vi "test -- PLL analyzer V1.vi"() -> ()   [LabVIEW 2017]
uses:
  lorentzian.ctl
  circle corners.ctl
  pid -- parameters.ctl
  <vilib>/event_ctls.llb/eventvkey.ctl
  cursor winow.ctl
  agregator -- action.ctl
  cursor window action.ctl
  four-corner circle transformation.ctl
  cursor action.ctl
  publisher action.ctl
  Q -- check range -- i -- real.vi
  draw a line.vi
  draw a circle.vi
  linear interpolation - real.vi
  linear interpolation iiii- complex.vi
  Q - not nan -- real.vi
  generate linear region.vi
panel:
  in  "all 3":enum32{"all", "other"}(tab)
  in  "total exp time (sec)":dbl=200.0 format="%#_10f"
  in  "total number of points":dbl=50000.0 format="%#_10f"
  out "dt (sec)":dbl=0.004 format="%#_10f"
  out "Plot: complex plane - filter":cluster{dbl[], dbl[]}[](graph)=[{[0.3333333333333333, 0.3330409433662861, 0.3321642864165014, 0.33070490043815925, 0.3286653456901683, 0.3260492002446019, 0.32286105370954366, 0.31910649917735573, 0.3147921234124937, 0.3099254952960838, 0.3045151525475336, 0.29857058674647097, 0.2921022266812878, 0.28512142005350216, 0.27764041357003316, 0.2696723314583158, 0.2612311524419466, 0.25233168521725213, 0.24298954247380383, 0.23322111350445518, 0.22304353545295275, 0.21247466324956327, 0.2015330382874583, 0.1902378558948106, 0.17860893165966557, 0.16666666666666669, 0.15443201170662058, 0.14192643052169093, 0.12917186215070103, 0.1161906824406051, 0.10300566479164915, 0.08963994020508864, 0.07611695670355195, 0.06246043819524158, 0.04869434285413729, 0.03484282108921789, 0.02093017317643784, 0.006980806627785684, -0.0069808066277855674, -0.020930173176437725, -0.034842821089217775, -0.0486943428541371, -0.062460438195241455, -0.07611695670355184, -0.08963994020508853, -0.10300566479164903, -0.116190682440605, -0.12917186215070092, -0.14192643052169077, -0.1544320117066205, -0.16666666666666657, -0.17860893165966546, -0.19023785589481051, -0.20153303828745828, -0.21247466324956313, -0.22304353545295263, -0.23322111350445507, -0.24298954247380378, -0.2523316852172521, -0.26123115244194656, -0.26967233145831576, -0.27764041357003305, -0.2851214200535021, -0.29210222668128777, -0.29857058674647086, -0.3045151525475336, -0.30992549529608376, -0.31479212341249363, -0.3191064991773557, -0.32286105370954366, -0.3260492002446018, -0.32866534569016825, -0.33070490043815925, -0.3321642864165014, -0.3330409433662861, -0.3333333333333333, -0.3330409433662861, -0.3321642864165014, -0.33070490043815925, -0.3286653456901683, -0.3260492002446019, -0.3228610537095437, -0.3191064991773558, -0.31479212341249374, -0.3099254952960838, -0.3045151525475337, -0.29857058674647097, -0.2921022266812879, -0.2851214200535023, -0.2776404135700333, -0.26967233145831593, -0.2612311524419467, -0.25233168521725224, -0.24298954247380392, -0.2332211135044552, -0.2230435354529528, -0.21247466324956338, -0.20153303828745844, -0.1902378558948107, -0.17860893165966568, -0.1666666666666668, -0.1544320117066207, -0.14192643052169096, -0.12917186215070106, -0.11619068244060515, -0.10300566479164919, -0.0896399402050886, -0.07611695670355222, -0.06246043819524183, -0.04869434285413747, -0.03484282108921807, -0.02093017317643803, -0.006980806627785872, 0.006980806627785453, 0.02093017317643761, 0.03484282108921766, 0.04869434285413707, 0.06246043819524142, 0.07611695670355181, 0.08963994020508849, 0.10300566479164908, 0.11619068244060474, 0.1291718621507007, 0.1419264305216906, 0.1544320117066203, 0.16666666666666644, 0.17860893165966532, 0.19023785589481038, 0.2015330382874581, 0.2124746632495631, 0.22304353545295258, 0.233221113504455, 0.24298954247380372, 0.252331685217252, 0.2612311524419465, 0.26967233145831576, 0.27764041357003294, 0.28512142005350205, 0.2921022266812877, 0.2985705867464708, 0.3045151525475335, 0.3099254952960837, 0.3147921234124936, 0.3191064991773557, 0.32286105370954366, 0.3260492002446018, 0.32866534569016825, 0.33070490043815925, 0.3321642864165014, 0.3330409433662861], [-0.3333333333333333, -0.31937478209026676, -0.30544071888922814, -0.2915555888118986, -0.27774375109463256, -0.2640294363940802, -0.2504367042783817, -0.23698940101850946, -0.2237111177538056, -0.21062514910510735, -0.1977544523080666, -0.1851216069383575, -0.17274877529942825, -0.16065766354228994, -0.148869483585552, -0.13740491590250895, -0.12628407324056323, -0.11552646533663152, -0.10515096469043711, -0.09517577345573225, -0.08561839150753528, -0.07649558574140364, -0.06782336065860123, -0.05961693028876536, -0.051890691499328345, -0.04465819873852045, -0.03793214025626174, -0.03172431584466018, -0.026045616137166494, -0.02090600350270283, -0.016314494568282156, -0.01227914440078065, -0.008807032375613255, -0.005904249757103797, -0.003575889012337241, -0.0018260348772422552, -0.000657757190576147, -7.310550838485197e-05, -7.310550838485197e-05, -0.000657757190576147, -0.0018260348772421997, -0.003575889012337241, -0.005904249757103741, -0.008807032375613255, -0.012279144400780595, -0.0163144945682821, -0.02090600350270283, -0.02604561613716644, -0.03172431584466012, -0.03793214025626174, -0.04465819873852045, -0.05189069149932829, -0.0596169302887653, -0.06782336065860123, -0.07649558574140353, -0.08561839150753517, -0.09517577345573214, -0.10515096469043705, -0.11552646533663147, -0.12628407324056315, -0.13740491590250892, -0.14886948358555185, -0.16065766354228977, -0.17274877529942811, -0.18512160693835739, -0.19775445230806651, -0.21062514910510727, -0.22371111775380553, -0.2369894010185093, -0.2504367042783816, -0.26402943639408005, -0.27774375109463245, -0.29155558881189847, -0.3054407188892281, -0.3193747820902667, -0.33333333333333315, -0.3472918845763997, -0.3612259477774383, -0.37511107785476794, -0.38892291557203396, -0.40263723027258636, -0.4162299623882848, -0.429677265648157, -0.4429555489128609, -0.45604151756155914, -0.4689122143585999, -0.481545059728309, -0.4939178913672383, -0.5060090031243767, -0.5177971830811146, -0.5292617507641575, -0.5403825934261033, -0.551140201330035, -0.5615157019762295, -0.5714908932109344, -0.5810482751591313, -0.5901710809252629, -0.5988433060080653, -0.6070497363779013, -0.6147759751673383, -0.6220084679281461, -0.6287345264104047, -0.6349423508220065, -0.6406210505295, -0.6457606631639639, -0.6503521720983845, -0.6543875222658859, -0.6578596342910533, -0.6607624169095627, -0.6630907776543293, -0.6648406317894244, -0.6660089094760905, -0.6665935611582818, -0.6665935611582818, -0.6660089094760905, -0.6648406317894244, -0.6630907776543293, -0.6607624169095629, -0.6578596342910534, -0.654387522265886, -0.6503521720983845, -0.6457606631639639, -0.6406210505295002, -0.6349423508220067, -0.628734526410405, -0.6220084679281463, -0.6147759751673385, -0.6070497363779015, -0.5988433060080656, -0.5901710809252632, -0.5810482751591315, -0.5714908932109346, -0.5615157019762296, -0.5511402013300353, -0.5403825934261035, -0.5292617507641577, -0.517797183081115, -0.506009003124377, -0.4939178913672387, -0.4815450597283094, -0.4689122143586003, -0.45604151756155953, -0.44295554891286126, -0.4296772656481574, -0.4162299623882851, -0.4026372302725866, -0.38892291557203423, -0.3751110778547682, -0.3612259477774386, -0.3472918845764]}, {[0.0, 0.0, 0.0, 0.0, 0.0, 0.0, 0.0, 0.0, 0.0, 0.0, 0.0, 0.0, 0.0, 0.0, 0.0, 0.0, 0.0, 0.0, 0.0, 0.0], [0.0, -0.03333333333333333, -0.06666666666666667, -0.1, -0.13333333333333333, -0.16666666666666666, -0.2, -0.23333333333333334, -0.26666666666666666, -0.3, -0.3333333333333333, -0.36666666666666664, -0.4, -0.43333333333333335, -0.4666666666666667, -0.5, -0.5333333333333333, -0.5666666666666667, -0.6, -0.6333333333333333]}, {[0.3333333333333333, 0.3, 0.26666666666666666, 0.2333333333333333, 0.19999999999999998, 0.16666666666666666, 0.1333333333333333, 0.09999999999999998, 0.06666666666666665, 0.033333333333333326, 0.0, -0.033333333333333326, -0.06666666666666671, -0.10000000000000003, -0.13333333333333336, -0.16666666666666669, -0.2, -0.23333333333333334, -0.26666666666666666, -0.3], [-0.3333333333333333, -0.3333333333333333, -0.3333333333333333, -0.3333333333333333, -0.3333333333333333, -0.3333333333333333, -0.3333333333333333, -0.3333333333333333, -0.3333333333333333, -0.3333333333333333, -0.3333333333333333, -0.3333333333333333, -0.3333333333333333, -0.3333333333333333, -0.3333333333333333, -0.3333333333333333, -0.3333333333333333, -0.3333333333333333, -0.3333333333333333, -0.3333333333333333]}]
  out "zi frreq":dbl=953.6192037473343 format="%#_5f"
  in  "PID parameters":T1={"P (sec)"=0.07054802310718643, "I (sec)"=0.2727272727272727}
  in  "visc hist time (sec)":dbl=5.0 format="%#_10f"
  out "dev frreq":dbl=952.9395994616418 format="%#_5f"
  out "off freq":dbl=0.6796042856924487 format="%#_5f"
  in  "I (sec)":dbl(slide)=0.2727272727272727 scale=0.0..3.0
  in  "P (sec)":dbl(slide)=0.07054802310718643 scale=0.001..1.0
  out "circle lorentzian":T2={"Amplitude"=1.0, "omega(0)"=1000.0, "Gamma"=3.0, "phase"=0.0, "Q"=300.0, "Norm  Ampl"=nan, "z (inf)"=0.0+0.0i, "4corners"={"z (-pi/2)"=9.277908004825974e-07+0.0007240755403629966i, "z(inf)"=2.6527949823343002e-05+0.0007477540585896028i, "z (pi/2)"=2.8494315967368497e-06+0.0007733542176124632i, "z center"=1.8886111986097237e-06+0.0007487148789877299i, "z(0)"=-2.2750727426123552e-05+0.000749675699385857i, "radius"=2.4658065287076567e-05}} {"z (inf)" format="%#9_9f"; "Q" format="%#9_9f"; "phase" format="%#9_9f"; "Gamma" format="%#9_9f"; "omega(0)" format="%#9_9f"}
  in  "cursor bracket: fit boundaries":T4={"left"=395.0, "right "=505.0, "center"=450.0, "window"=110.0, "cursors"=[0, 1, 2], "relative"=0, "absolute"=0, "fixed vertical offset"=0.0, "vertical offset"=0.0, "skew"=0.0, "default window frac"=0.1, "kind"=enum."symmetric", "skew.left"=0.5, "skew.right"=0.5, "Plot ref"=refnum, "wing order"=enum."forw"}
  out "VKey":T5=enum."Cmd"
  out "Char":i16
  in  "lorentzian -- basic":T2={"Amplitude"=1.0, "omega(0)"=1000.0, "Gamma"=3.0, "phase"=0.0, "Q"=300.0, "Norm  Ampl"=nan, "z (inf)"=0.0+0.0i, "4corners"={"z (-pi/2)"=9.277908004825974e-07+0.0007240755403629966i, "z(inf)"=2.6527949823343002e-05+0.0007477540585896028i, "z (pi/2)"=2.8494315967368497e-06+0.0007733542176124632i, "z center"=1.8886111986097237e-06+0.0007487148789877299i, "z(0)"=-2.2750727426123552e-05+0.000749675699385857i, "radius"=2.4658065287076567e-05}} {"z (inf)" format="%#9_9f"; "Q" format="%#9_9f"; "phase" format="%#9_9f"; "Gamma" format="%#9_9f"; "omega(0)" format="%#9_9f"}
  in  "all 2":enum32{"all", "other"}(tab)
  out "Plot: circle sweep window":cluster{dbl[], dbl[]}[](graph)
  out "dev out":cdb=0.2506043041344095-0.553125493931521i format="%#_10f"
  out "time(sec)":dbl=179.1847980649909 format="%#_5f"
  in  "all":enum32{"all", "other"}(tab)
  out "Plot: hist":cluster{"all rows":dbl[], "all rows":dbl[]}[](graph)
  out "center freq (Hz)":dbl=-0.35260838541595674
  out "window  (Hz)":dbl=17.234446484426172
  out "left freq (Hz)":dbl=-8.969831627629043
  out "right freq (Hz)":dbl=8.26461485679713
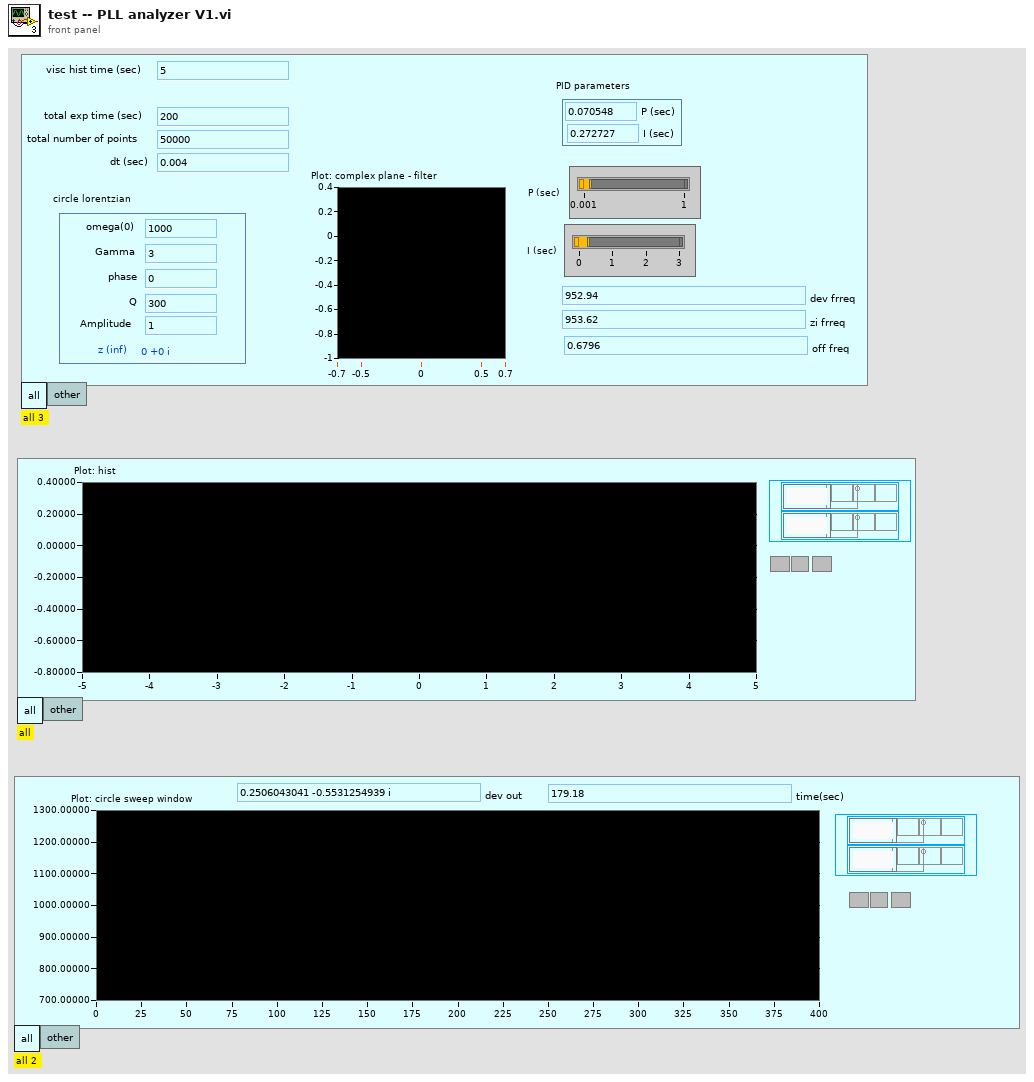
[diagram p1: front panel]
types:
  T1 = typedef "pid -- parameters.ctl" = cluster{"P (sec)":dbl, "I (sec)":dbl}
  T2 = typedef "lorentzian.ctl" = cluster{"Amplitude":dbl, "omega(0)":dbl, "Gamma":dbl, "phase":dbl, "Q":dbl, "Norm  Ampl":dbl, "z (inf)":cdb, "4corners":T3}
  T3 = typedef "circle corners.ctl" = cluster{"z (-pi/2)":cdb, "z(inf)":cdb, "z (pi/2)":cdb, "z center":cdb, "z(0)":cdb, "radius":dbl}
  T4 = typedef "cursor winow.ctl" = cluster{"left":dbl, "right ":dbl, "center":dbl, "window":dbl, "cursors":i32[], "relative":i32, "absolute":i32, "fixed vertical offset":dbl, "vertical offset":dbl, "skew":dbl, "default window frac":dbl, "kind":enum16{"symmetric", "skewed", "fancy"}, "skew.left":dbl, "skew.right":dbl, "Plot ref":refnum<vi>, "wing order":enum16{"forw", "back"}}
  T5 = typedef "eventvkey.ctl" = enum16{"ASCII", "Enter", "Return", "Shift", "Ctrl", "Alt", "Cmd", "Opt", "Caps", "NumLock", "Clear", "Break", "Up", "Down", "Left", "Right", "Insert", "Delete", "Home", "End", "PageUp", "PageDown", "Escape", "Help", "Pause", "ScrollLock", "F1", "F2", "F3", "F4", "F5", "F6", "F7", "F8", "F9", "F10", "F11", "F12", "F13", "F14", "F15", "F16", "F17", "F18", "F19", "F20", "F21", "F22", "F23", "F24", "Play", "VolumeUp", "VolumeDown", "Mute", "Two Byte Char"}
  T6 = typedef "cursor window action.ctl" = enum16{"balance", "h. offset change", "cursor moves", "change center", "change window", "init", "check", "reset", "set y to middle", "idle", "-write all Y", "-write left.X", "-write center.X", "-write right.X", "-write all X", "-change center", "-change window", "-change skew", "-read cursor 2", "-read cursor 1", "-read cursor 0", "-read all cursors", "-reset", "-read plot scale", "-set y to middle", "-Q: center.Y is visible", "-Q: window is visible", "-parse center.Y", "-right left from center", "-left move", "-right move", "-set center.Y", "-empty", "-set cursors to default", "-check", "-write center.Y", "-copy cursor 1", "-copy cursor 0", "-copy cursor 2", "move right", "move left", "shrink", "broaden", "skew up", "skew down", "-write plot scale", "zoom X", "change cen&win", "zoom to all data", "color--red", "color--green", "color--yellow", "read", "zoom out", "zoom in", "slide right", "slide left"}
  T7 = typedef "agregator -- action.ctl" = enum16{"append", "interpolate", "empty!", "force", "init", "scale", "read last"}
  T8 = typedef "publisher action.ctl" = enum16{"set", "get"}
  T9 = typedef "cursor action.ctl" = enum16{"range", "read", "write", "check", "zoom out", "smart zoom out"}
  T10 = typedef "four-corner circle transformation.ctl" = enum16{"z(c) z(inf)", "z(c) z(zero)", "fix phase", "calculate lorentzian", "z(0) z(+-pi/2)", "shift to zcenter", "to  canonical", "get canonical phase", "get4corners"}
  T11 = typedef "interpolation state - complex.ctl" = cluster{"requested size":i32, "Array":cdb[], "actual number of elements":i32}
  T12 = typedef "interpolation state - real.ctl" = cluster{"requested size":i32, "Array":dbl[], "actual number of elements":i32}
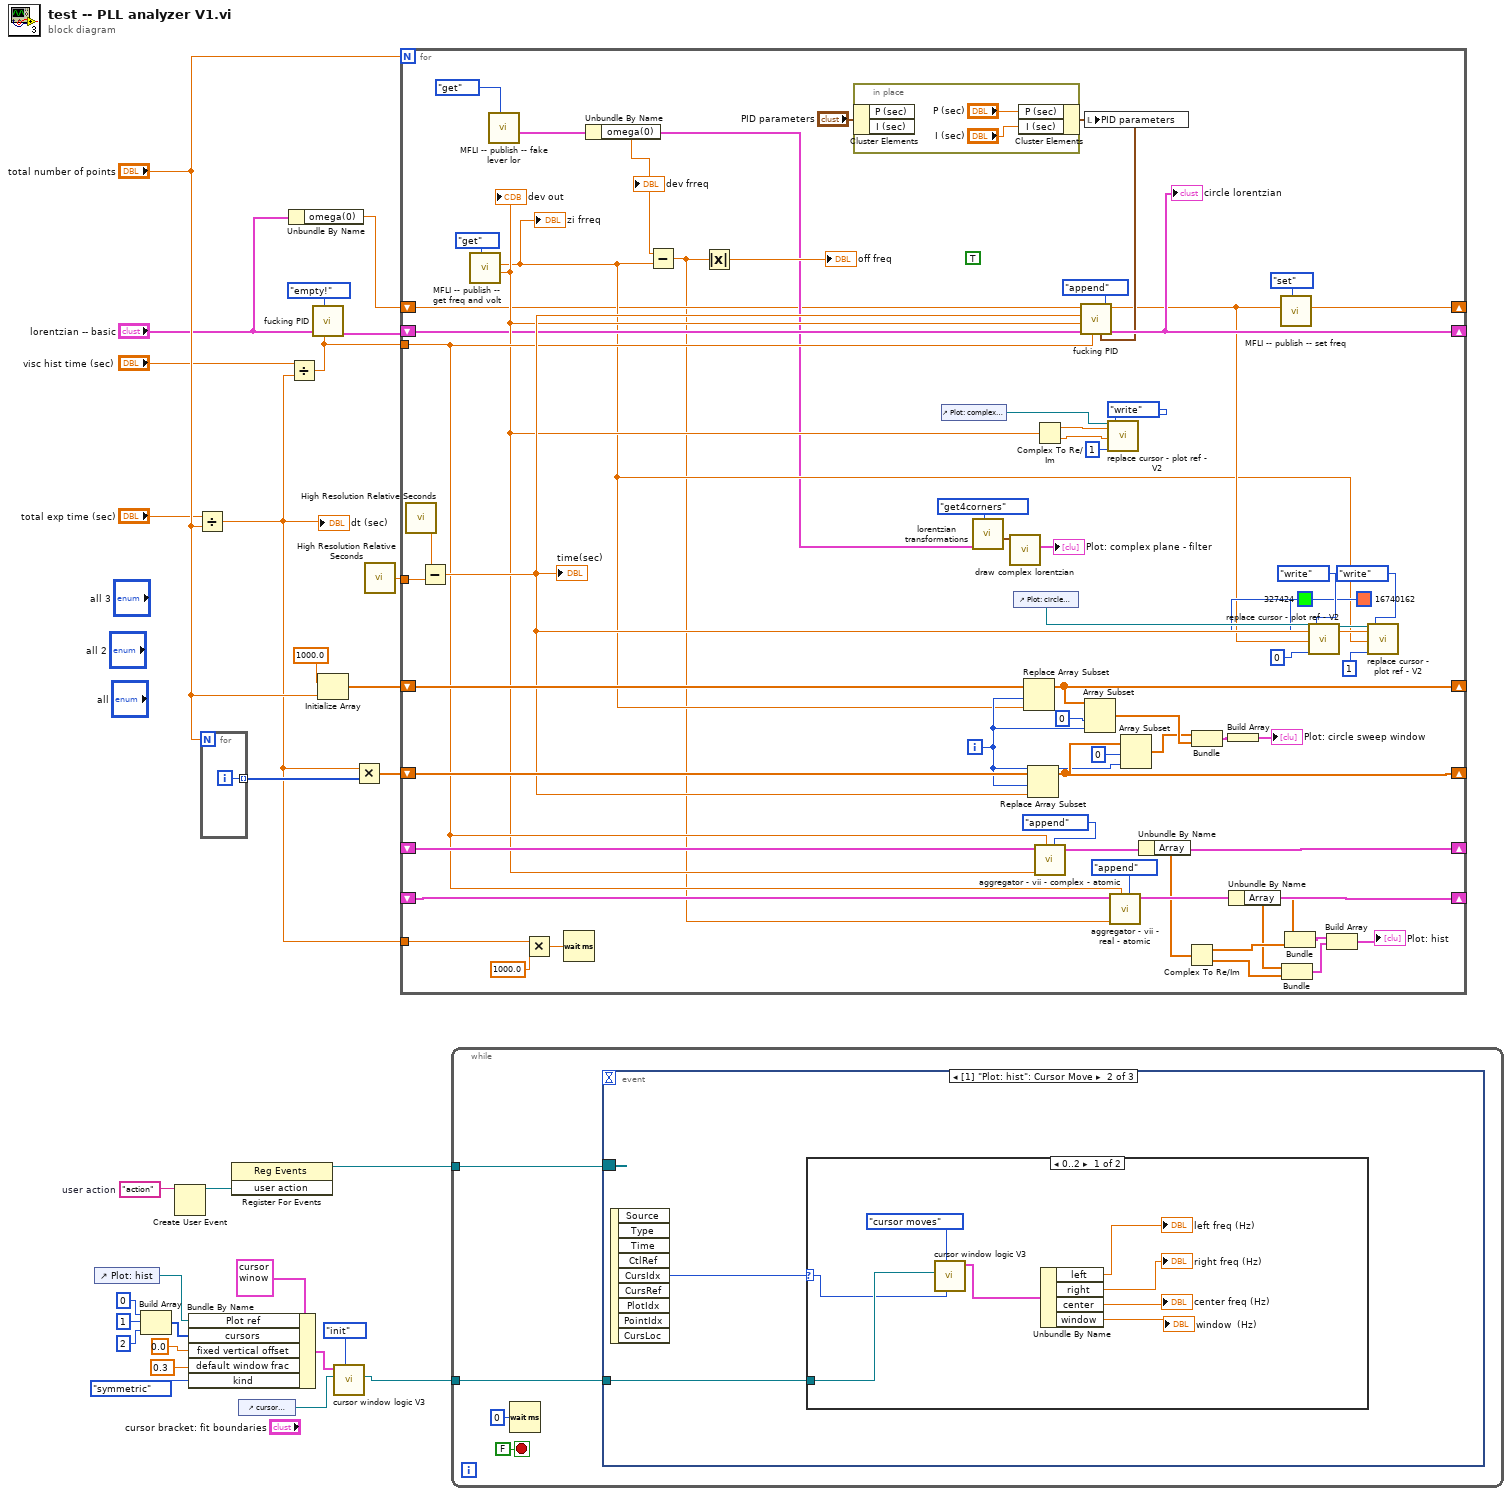
[diagram p0: block diagram]
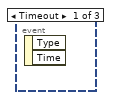
[diagram p2: hidden frame]
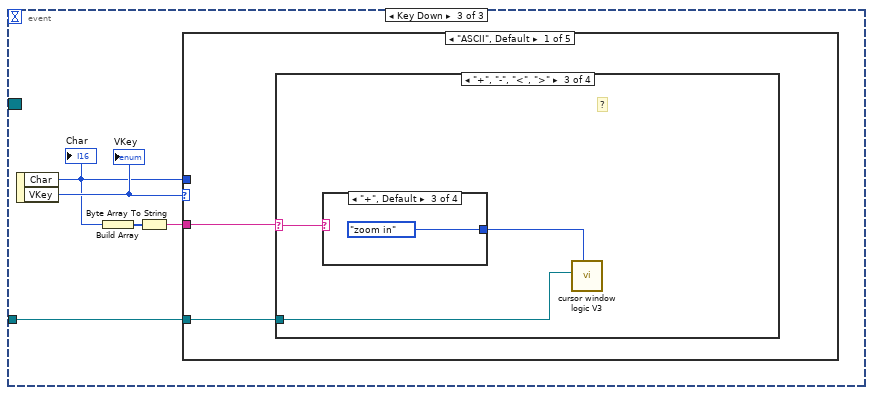
[diagram p4: hidden frame]
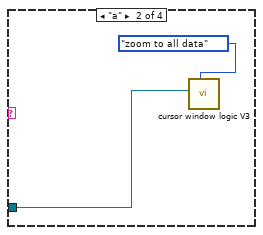
[diagram p6: hidden frame]
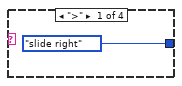
[diagram p7: hidden frame]
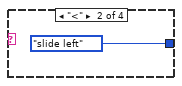
[diagram p8: hidden frame]
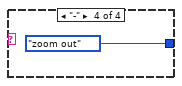
[diagram p9: hidden frame]
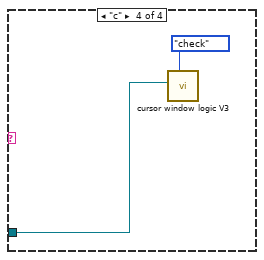
[diagram p10: hidden frame]
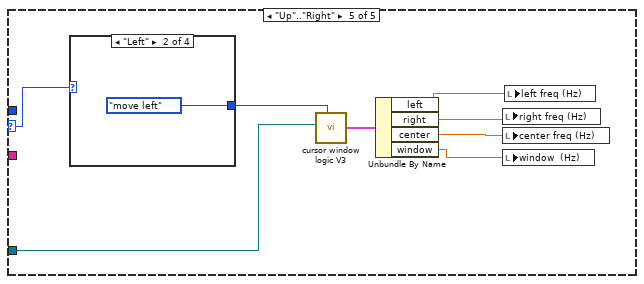
[diagram p14: hidden frame]
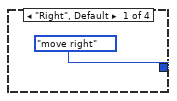
[diagram p15: hidden frame]
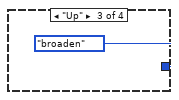
[diagram p16: hidden frame]
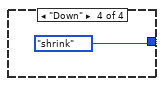
[diagram p17: hidden frame]
diagram:
  w18 = "action"  # user action
  n1 = control-ref of="Plot: hist"() -> (w16:refnum<vi>)
  n2 = Build Array(0, 1, 2) -> (w5:i32[])
  n3 = Create User Event(user event datatype=w18) -> (user event=w19:refnum<user-event>)  [unwired: 1 in, 1 out]
  n4 = Bundle By Name(cluster=T4 {"left"=0.0, "right "=0.0, "center"=0.0, "window"=0.0, "cursors"=[], "relative"=0, "absolute"=0, "fixed vertical offset"=0.0, "vertical offset"=0.0, "skew"=0.0, "default window frac"=0.0, "kind"=enum."symmetric", "skew.left"=0.0, "skew.right"=0.0, "Plot ref"=refnum, "wing order"=enum."forw"} ("cursor bracket: All, data window"), "Plot ref"=w16, "cursors"=w5, "fixed vertical offset"=0.0, "default window frac"=0.3 ("fixed vertical offset"), "kind"=enum16{"symmetric", "skewed", "fancy"}."symmetric") -> (w13:T4)
  n5 = Divide(x="total exp time (sec)", y="total number of points") -> (x/y=w24:dbl)
  "dt (sec)" <- w24
  n6 = for {
    N: "total number of points" -> [_]
    tunnel: [w31] -> w26 mode=indexing
    i -> [w31]
  }
  n7 = register-events(w19) -> (reference out=w17:refnum<event-registration>)  [unwired: 2 in, 1 out]
  n8 = control-ref of="cursor bracket: fit boundaries"() -> (w15:refnum<vi>)
  n9 = Unbundle By Name("lorentzian -- basic") -> ("omega(0)"=w1:dbl)
  n10 = Divide(x="visc hist time (sec)", y=w24) -> (x/y=w21:dbl)
  n11 = call "fucking PID.vi"("requested size"=w21, "PID action"=agregator_--_action."empty!", "lorentzian IN"="lorentzian -- basic") -> ("lorentzian  OUT"=w3:T2)  [unwired: 5 in, 3 out]
  n12 = Initialize Array(1000.0, "total number of points") -> (w29:dbl[])
  n13 = call "cursor window logic V3.vi"("cursor window action"=cursor_window_action."init", "cursor window in"=w15, "cursor window init"=w13) -> ("cursor window out"=w20:refnum<vi>)  [unwired: 7 in, 1 out]
  n14 = Multiply(x=w24, y=w26) -> (x*y=w25:dbl[])
  n15 = call <vilib>:"High Resolution Relative Seconds.vi"() -> ("relative seconds"=w30:dbl)
  n16 = for {
    N: "total number of points" -> [_]
    tunnel: w30 -> [w95]
    shift-right: [w73] -> _
    shift-left: w29 -> [w94]
    shift-right: [w69] -> _
    shift-left: w25 -> [w93]
    tunnel: w24 -> [w90]
    tunnel: w21 -> [w51]
    shift-right: [w62] -> _
    shift-left: w3 -> [w39]
    shift-right: [w47] -> _
    shift-left: _ -> [w55]
    shift-right: [w49] -> _
    shift-left: _ -> [w52]
    shift-right: [w34] -> _
    shift-left: w1 -> [w33]
    i -> [w67]
    (unwired) TRUE
    n17 = call <vilib>:"High Resolution Relative Seconds.vi"() -> ("relative seconds"=w92:dbl)
    n18 = Subtract(x=w92, y=w95) -> (x-y=w65:dbl)
    "time(sec)" <- w65
    n19 = call "MFLI -- publish -- get freq and volt.vi"("publisher action"=publisher_action."get") -> ("Voltage out (V)"=w42:cdb, "freq out (Hz)"=w38:dbl)  [unwired: 9 in]
    "dev out" <- w42
    "zi frreq" <- w38
    n20 = call "MFLI -- publish -- fake lever lor.vi"("publisher action"=publisher_action."get") -> ("lorentzian OUT"=w35:T2)  [unwired: 10 in]
    n21 = Multiply(x=w90, y=1000.0) -> (x*y=w91:dbl)
    n22 = Wait (ms)(milliseconds to wait=w91) -> ()  [unwired: 1 out]
    n23 = Unbundle By Name(w35) -> ("omega(0)"=w36:dbl)
    "dev frreq" <- w36
    n24 = Subtract(x=w36, y=w38) -> (x-y=w32:dbl)
    n25 = Absolute Value(x=w32) -> (abs(x)=→"off freq":dbl)
    n26 = in-place {
      n27 = in-place-cluster #1("PID parameters") -> ()  [unwired: 2 out]
      n28 = in-place-cluster #1("P (sec)"="P (sec)", "I (sec)"="I (sec)") -> (w44:T1)
    }
    n29 = control-ref of="Plot: complex plane - filter"() -> (w81:refnum<vi>)
    n30 = call "lorentzian transformations.vi"("4 corner circle transformation"=four-corner_circle_transformation."get4corners", "lorentzian in"=w35) -> ("4corners our"=w88:T3)  [unwired: 7 in, 2 out]
    n31 = call "draw complex lorentzian.vi"("4 corners"=w88) -> ("fancy circles"=→"Plot: complex plane - filter":cluster{dbl[], dbl[]}[])  [unwired: 10 in]
    n32 = control-ref of="Plot: circle sweep window"() -> (w74:refnum<vi>)
    n33 = Replace Array Subset(array=w94, new element=w38, index=w67) -> (w73:dbl[])
    n34 = Replace Array Subset(array=w93, new element=w65, index=w67) -> (w69:dbl[])
    n35 = Complex To Re/Im(x + iy=w42) -> (x=w83:dbl, y=w82:dbl)
    n36 = call "aggregator - vii - complex - atomic.vi"("aggregator action"=agregator_--_action."append", "requested size"=w51, "number"=w42, "state IN"=w55) -> ("state OUT"=w47:T11)  [unwired: 4 in, 3 out]
    n37 = call "fucking PID.vi"("PID parameters"=w44, "requested size"=w51, "PID action"=agregator_--_action."append", "lorentzian IN"=w39, "voltage IN (V)"=w42, "time in (sec)"=w65, "frequency IN (Hz)"=w33) -> ("lorentzian  OUT"=w62:T2, "frequency out (Hz)"=w40:dbl)  [unwired: 1 in, 2 out]
    "circle lorentzian" <- w62
    n38 = local write "PID parameters"(w44) -> ()
    n39 = Array Subset(array=w73, index=0 ("cursor index"), length=w67) -> (w71:dbl[])
    n40 = call "replace cursor - plot ref - V2.vi"("Plot ref in"=w81, "new X"=w83, "new  Y"=w82, "cursor index"=1, "cursor action"=cursor_action."write") -> ()  [unwired: 12 in, 3 out]
    n41 = call "aggregator - vii - real - atomic.vi"("aggregator action"=agregator_--_action."append", "requested size"=w51, "number"=w32, "state IN"=w52) -> ("state OUT"=w49:T12)  [unwired: 4 in, 3 out]
    n42 = Array Subset(array=w69, index=0 ("cursor index"), length=w67) -> (w70:dbl[])
    n43 = Unbundle By Name(w47) -> ("Array"=w46:cdb[])
    n44 = Complex To Re/Im(x + iy=w46) -> (x=w60:dbl[], y=w59:dbl[])
    n45 = Bundle(w70, w71) -> (w79:cluster{dbl[], dbl[]})  [unwired: 1 in]
    n46 = Build Array(w79) -> (→"Plot: circle sweep window":cluster{dbl[], dbl[]}[])
    n47 = Unbundle By Name(w49) -> ("Array"=w48:dbl[])
    n48 = call "MFLI -- publish -- set freq.vi"("publisher action"=publisher_action."set", "freq IN (Hz)"=w40) -> ("freq out (Hz)"=w34:dbl)  [unwired: 9 in]
    n49 = Bundle("Array"=w48, w59) -> (w57:cluster{"Array":dbl[], dbl[]})  [unwired: 1 in]
    n50 = Bundle("Array"=w48, w60) -> (w58:cluster{"Array":dbl[], dbl[]})  [unwired: 1 in]
    n51 = call "replace cursor - plot ref - V2.vi"("Plot ref in"=w74, "new X"=w65, "new  Y"=w40, "cursor index"=0, "cursor action"=cursor_action."write", "Color Box"=u32 327424) -> ("Plot ref out"=w66:refnum<vi>)  [unwired: 11 in, 2 out]
    n52 = Build Array(w58, w57) -> (→"Plot: hist":cluster{"Array":dbl[], dbl[]}[])
    n53 = call "replace cursor - plot ref - V2.vi"("Plot ref in"=w66, "new X"=w65, "new  Y"=w38, "cursor index"=1, "cursor action"=cursor_action."write", "Color Box"=u32 16740162) -> ()  [unwired: 11 in, 3 out]
  }
  n54 = while {
    tunnel: w17 -> [w101]
    tunnel: w20 -> [w99]
    stop <- FALSE stop-if-true
    n55 = Wait (ms)(milliseconds to wait=u32 0) -> ()  [unwired: 1 out]
    n56 = event shown="[1] \"Plot: hist\": Cursor Move" {
      selector: w101 -> [_ _ _]
      dyn-events: _ -> [_ _ _]
      timeout: _ -> [_ _ _]
      tunnel: w99 -> [_ w103 w112]
      event Timeout {
        n57 = event-data() -> ()  [unwired: 1 in, 2 out]
      }
      event "Plot: hist": Cursor Move {
        n58 = event-data() -> ("CursIdx"=w102:i32)  [unwired: 1 in, 8 out]
        n59 = case shown="0..2" w102 {
          selector: w102 -> [w109 _]
          tunnel: w103 -> [w111 _]
          frame 0..2 {
            n60 = call "cursor window logic V3.vi"("CursIdx"=w109, "cursor window action"=cursor_window_action."cursor moves", "cursor window in"=w111) -> ("cursor window out"=w108:T4)  [unwired: 7 in, 1 out]
            n61 = Unbundle By Name(w108) -> ("left"=→"left freq (Hz)":dbl, "right"=→"right freq (Hz)":dbl, "center"=→"center freq (Hz)":dbl, "window"=→"window  (Hz)":dbl)
          }
          frame 3, Default {
          }
        }
      }
      event Key Down {
        n62 = event-data() -> ("Char"=w114:i16, "VKey"=w116:T5)  [unwired: 1 in]
        "Char" <- w114
        "VKey" <- w116
        n63 = Build Array(w114) -> (w115:i16[])
        n64 = Byte Array To String(unsigned byte array=w115) -> (string=w113:string)
        n65 = case shown="\"ASCII\", Default" w116 {
          selector: w116 -> [_ _ _ _ w137]
          tunnel: w114 -> [_ _ _ _ _]
          tunnel: w113 -> [w118 _ _ _ _]
          tunnel: w112 -> [w117 _ _ _ w130]
          frame "ASCII", Default {
            n66 = case shown="\"+\", \"-\", \"<\", \">\"" w118 {
              selector: w118 -> [_ _ w122 _]
              tunnel: w117 -> [_ w119 w123 w128]
              frame "0", Default {
              }
              frame "a" {
                n67 = call "cursor window logic V3.vi"("cursor window action"=cursor_window_action."zoom to all data", "cursor window in"=w119) -> ()  [unwired: 8 in, 2 out]
              }
              frame "+", "-", "<", ">" {
                # "?"
                n68 = case shown="\"+\", Default" w122 {
                  tunnel: [cursor_window_action."slide right" ("cursor window action") cursor_window_action."slide left" ("cursor window action") cursor_window_action."zoom in" ("cursor window action") cursor_window_action."zoom out" ("cursor window action")] -> w121
                  frame ">" {
                  }
                  frame "<" {
                  }
                  frame "+", Default {
                  }
                  frame "-" {
                  }
                }
                n69 = call "cursor window logic V3.vi"("cursor window action"=w121, "cursor window in"=w123) -> ()  [unwired: 8 in, 2 out]
              }
              frame "c" {
                n70 = call "cursor window logic V3.vi"("cursor window action"=cursor_window_action."check", "cursor window in"=w128) -> ()  [unwired: 8 in, 2 out]
              }
            }
          }
          frame "Escape" {
          }
          frame "PageUp" {
          }
          frame "PageDown" {
          }
          frame "Up".."Right" {
            n71 = case shown="\"Left\"" w137 {
              tunnel: [cursor_window_action."move right" ("cursor window action") cursor_window_action."move left" ("cursor window action") cursor_window_action."broaden" ("cursor window action") cursor_window_action."shrink" ("cursor window action")] -> w132
              frame "Right", Default {
              }
              frame "Left" {
              }
              frame "Up" {
              }
              frame "Down" {
              }
            }
            n72 = call "cursor window logic V3.vi"("cursor window action"=w132, "cursor window in"=w130) -> ("cursor window out"=w131:T4)  [unwired: 8 in, 1 out]
            n73 = Unbundle By Name(w131) -> ("left"=w136:dbl, "right"=w135:dbl, "center"=w134:dbl, "window"=w133:dbl)
            n74 = local write "right freq (Hz)"(w135) -> ()
            n75 = local write "center freq (Hz)"(w134) -> ()
            n76 = local write "window  (Hz)"(w133) -> ()
            n77 = local write "left freq (Hz)"(w136) -> ()
          }
        }
      }
    }
  }
